vi "ProcessPedCalDataV1729A.vi"(9 "# Events to Avg":i32=100, 10 "Data In":u32[][](array[numeric]), 11 "Offset":i16) -> (1 "Channel Data":dbl[][](array[numeric]))   [LabVIEW 2014]
panel:
  out "Wfm Plot":dbl[][](graph)
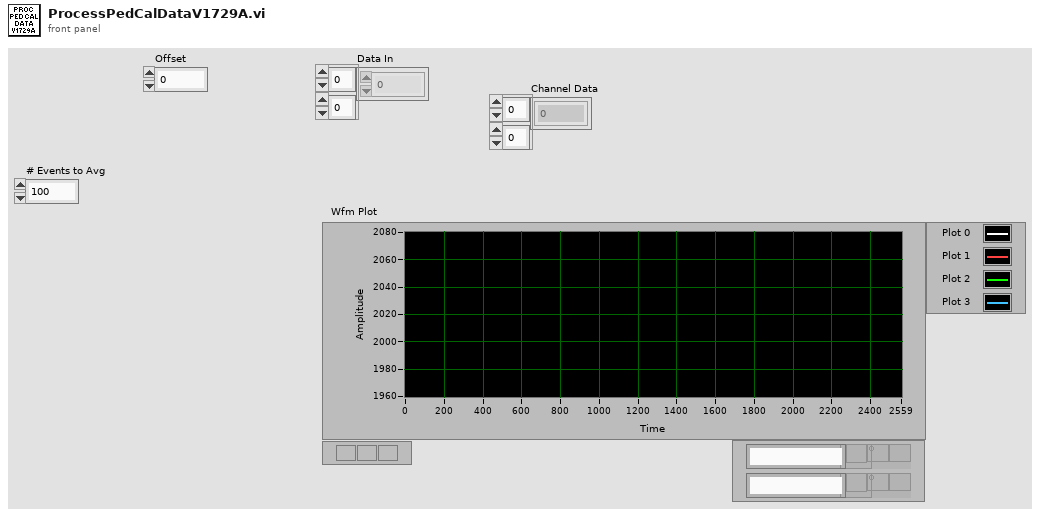
[diagram p1: front panel]
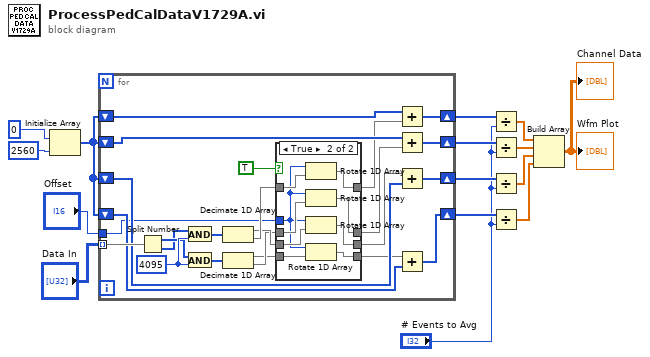
[diagram p0: block diagram]
diagram:
  n1 = Initialize Array(u32 0 ("element"), 2560 ("dimension size")) -> (w12:u32[])
  n2 = for {
    tunnel: "Data In" -> [w34] mode=indexing
    shift-right: [w33] -> w9
    shift-left: w12 -> [w32]
    shift-right: [w31] -> w8
    shift-left: w12 -> [w30]
    shift-right: [w29] -> w10
    shift-left: w12 -> [w28]
    shift-right: [w27] -> w11
    shift-left: w12 -> [w26]
    tunnel: "Offset" -> [w18]
    w39 = u16 4095 ("Numeric")
    n3 = Split Number(x=w34) -> (hi(x)=w38:u16[], lo(x)=w37:u16[])
    n4 = And(x=w37, y=w39) -> (x .and. y?=w36:u16[])
    n5 = And(x=w38, y=w39) -> (x .and. y?=w35:u16[])
    n6 = Decimate 1D Array(w36) -> (w23:u16[], w25:u16[])
    n7 = Decimate 1D Array(w35) -> (w19:u16[], w21:u16[])
    n8 = case shown="True" TRUE {
      tunnel: w25 -> [w40 w52]
      tunnel: [w40 w51] -> w24
      tunnel: w23 -> [w41 w50]
      tunnel: [w41 w49] -> w22
      tunnel: w21 -> [w42 w48]
      tunnel: [w42 w47] -> w20
      tunnel: w19 -> [w43 w46]
      tunnel: w18 -> [_ w45]
      tunnel: [w43 w44] -> w17
      frame False {
      }
      frame True {
        n9 = Rotate 1D Array(1:w52, 2:w45) -> (0:w51:u16[])
        n10 = Rotate 1D Array(1:w48, 2:w45) -> (0:w47:u16[])
        n11 = Rotate 1D Array(1:w50, 2:w45) -> (0:w49:u16[])
        n12 = Rotate 1D Array(1:w46, 2:w45) -> (0:w44:u16[])
      }
    }
    n13 = Add(x=w32, y=w24) -> (x+y=w33:u32[])
    n14 = Add(x=w30, y=w20) -> (x+y=w31:u32[])
    n15 = Add(x=w22, y=w28) -> (x+y=w29:u32[])
    n16 = Add(x=w17, y=w26) -> (x+y=w27:u32[])
  }
  n17 = Divide(x=w9, y="# Events to Avg") -> (x/y=w4:dbl[])
  n18 = Divide(x=w8, y="# Events to Avg") -> (x/y=w3:dbl[])
  n19 = Divide(x=w10, y="# Events to Avg") -> (x/y=w5:dbl[])
  n20 = Divide(x=w11, y="# Events to Avg") -> (x/y=w6:dbl[])
  n21 = Build Array(w4, w3, w5, w6) -> (→"Wfm Plot" →"Channel Data":dbl[][])
